vi "To JSON Tree.vi"(8 "error in (no error)":errorcluster, 11 "error in":refnum<class "error.lvclass">) -> (0 "error out":errorcluster, 2 "JSON Tree Out":variant, 3 "error out":refnum<class "error.lvclass">)   [LabVIEW 2015, in "error.lvclass"]
uses:
  error.lvclass
  error.lvclass/error.ctl
  <vilib>/NI/i3 JSON/JSON Generation/Create Value Files/Create Value - Object.vi
  <vilib>/NI/i3 JSON/JSON Generation/Add Object Parameter Files/Add Object Parameter - Numeric.vi
  <vilib>/NI/i3 JSON/JSON Generation/Add Object Parameter Files/Add Object Parameter - String.vi
  <vilib>/NI/i3 JSON/JSON Generation/Add Object Parameter Files/Add Object Parameter - Known Type.vi
  <vilib>/NI/i3 JSON/i3-json.lvlib
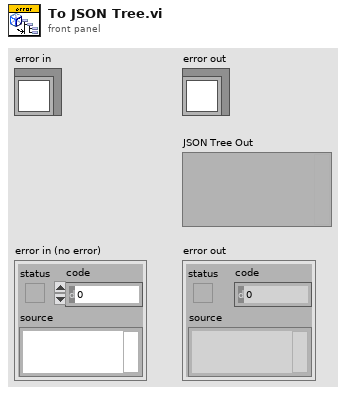
[diagram p1: front panel]
types:
  T1 = typedef "i3-json.lvlib/JSON Type.ctl" = enum8{"JSON Compatible", "JSON Array", "JSON Object", "JSON Null", "Double", "String", "Boolean", "Unknown"}
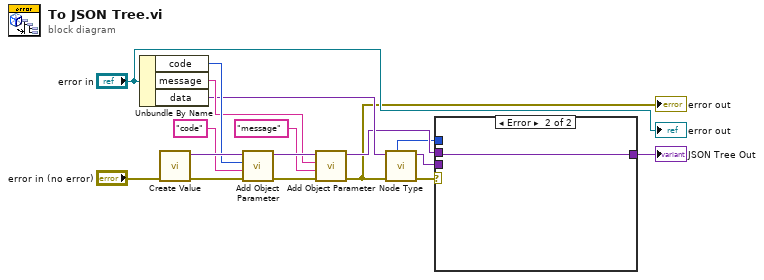
[diagram p0: block diagram]
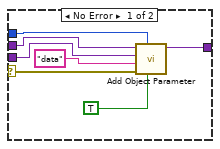
[diagram p2: hidden frame]
diagram:
  n1 = Unbundle By Name("error in") -> ("code"=w15:i32, "message"=w12:string, "data"=w10:variant)
  n2 = call-poly <vilib>:"Create Value.vi"("error in (no error)"="error in (no error)") -> ("error out"=w5:errorcluster, "JSON Tree"=w16:variant)  [unwired: 9 in]
  n3 = call-poly <vilib>:"Add Object Parameter.vi"("error in (no error)"=w5, "Name"="code", "Numeric"=w15, "JSON Tree in (JSON Object)"=w16) -> ("error out"=w4:errorcluster, "JSON Tree out (JSON Object)"=w13:variant)  [unwired: 6 in]
  n4 = call-poly <vilib>:"Add Object Parameter.vi"("error in (no error)"=w4, "Name"="message", "String"=w12, "JSON Tree in (JSON Object)"=w13) -> ("error out"=w3:errorcluster, "JSON Tree out (JSON Object)"=w9:variant)  [unwired: 6 in]
  "error out" <- w3
  n5 = call <vilib>:"Node Type.vi"("error in (no error)"=w3, "JSON Tree In"=w10) -> ("error out"=w2:errorcluster, "JSON Tree Out"=w1:variant, "JSON Type"=w8:T1)  [unwired: 5 in, 2 out]
  n6 = case shown="Error" w2 {
    selector: w2 -> [w18 _]
    tunnel: w9 -> [w24 w25]
    tunnel: w8 -> [w23 _]
    tunnel: w1 -> [w22 _]
    tunnel: [w20 w25] -> w7
    frame No Error {
      n7 = call-poly <vilib>:"Add Object Parameter.vi"("Add Parameter as JSON Tree?"=TRUE, "JSON Type"=w23, "error in (no error)"=w18, "Name"="data", "Value"=w22, "JSON Tree in (JSON Object)"=w24) -> ("JSON Tree out (JSON Object)"=w20:variant)  [unwired: 4 in, 1 out]
    }
    frame Error {
    }
  }
  "JSON Tree Out" <- w7
  "error out" <- "error in"
